vi "dat_muxed_thermistors.vi"() -> (20 "v_piston_0":fxp<+/-,24,5>, 21 "v_piston_1":fxp<+/-,24,5>, 22 "v_piston_2":fxp<+/-,24,5>, 23 "v_piston_3":fxp<+/-,24,5>, 24 "v_piston_4":fxp<+/-,24,5>, 25 "v_piston_5":fxp<+/-,24,5>, 26 "v_piston_6":fxp<+/-,24,5>, 27 "v_piston_7":fxp<+/-,24,5>)   [LabVIEW 2018]
uses:
  <vilib>/rvi/DataTransferAndStorage/Container/Common/niFpgaContainerExecOnDevCompGetState.vi
  <vilib>/rvi/Emulation/niFpgaEmulationIsFPGAContextNoSignature.vi
  <vilib>/rvi/Emulation/niFpgaSctlEmulationGetInTimedLoop.vi
  <vilib>/rvi/errors/niFpgaSetErrorForExecOnDevCompSimple.vi
  <vilib>/rvi/eio/common/nirviEmuReportErrorAndStop.vi
  <vilib>/rvi/DataTransferAndStorage/Container/Common/niFpgaContainerGetUniqueNameForEmu.vi
  <vilib>/rvi/FIFO/Fifo_Resource/nirvififoEmulationSetSize.vi
  <vilib>/rvi/FIFO/Fifo_Resource/nirviFifoEmulationQueueMgr.vi
  <instcachedir>/0/nirviFifoEmulationQueueMgr_E5CAEC123FF24DC58D834DCA3CDAA9B5.lvgen/nirviFifoEmulationQueueMgr_E5CAEC123FF24DC58D834DCA3CDAA9B5_003.vi
  <vilib>/rvi/FIFO/Fifo_Resource/nirvififoEmulationDetermineInputValidOut.vi
  <vilib>/rvi/FIFO/Fifo_Resource/nirvififoEmulationCreateLock.vi
  <vilib>/rvi/Emulation/niFpgaProcessEmulError.vi
  <vilib>/rvi/FIFO/Fifo_Resource/nirvififoEmulationObtainLock.vi
  <vilib>/rvi/FIFO/Fifo_Resource/nirvififoEmulationReleaseLock.vi
  <vilib>/rvi/occurrence/nirviWaitOnOccurrenceBase.vi
  <vilib>/rvi/errors/nirviReportUnexpectedCaseInternalError.vi
  <vilib>/rvi/errors/nirviReportUnexpectedCaseInternalError (U32).vi
  <vilib>/Utility/error.llb/Clear Errors.vi
  <vilib>/rvi/interface/RandomDataEmulation/niFpgaRandomDataHandleErrors.vi
  <vilib>/rvi/DataTransferAndStorage/Container/XNode/niFpgaContainer.xnode
  <vilib>/rvi/FIFO/Fifo_Resource/niFpgaFifoEmulationRefIn.vi
types:
  T1 = cluster{"Analog":fxp<+/-,24,5>, "Index":fxp<+,3,3>}
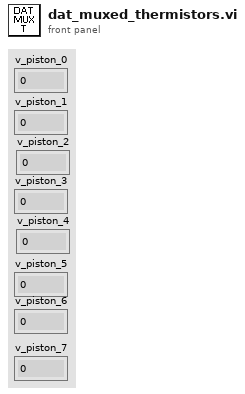
[diagram p1: front panel]
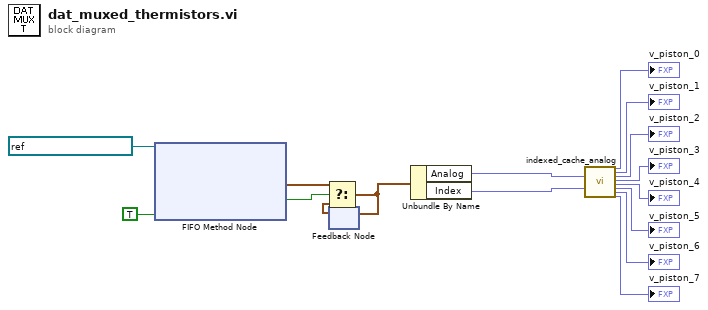
[diagram p0: block diagram]
diagram:
  n1 = xnode ("FIFO Method Node")("Ready for Output"=TRUE, "FIFO In"=refnum<k21> "T_pistons_indexed") -> ("Element"=w3:T1, "Output Valid"=w4:bool)  [unwired: 1 out]
  n2 = feedback #1() -> (w1:T1)  [unwired: 1 in]
  n3 = Select(t=w3, s=w4, f=w1) -> (s? t:f=w2:T1)
  n4 = feedback-in #1(w2) -> ()
  n5 = Unbundle By Name(w2) -> ("Analog"=w16:fxp<+/-,24,5>, "Index"=w15:fxp<+,3,3>)
  n6 = call "indexed_cache_analog.vi"("new_val"=w16, "index"=w15) -> ("$val_0"=→"v_piston_0":fxp<+/-,24,5>, "$val_1"=→"v_piston_1":fxp<+/-,24,5>, "$val_2"=→"v_piston_2":fxp<+/-,24,5>, "$val_3"=→"v_piston_3":fxp<+/-,24,5>, "$val_4"=→"v_piston_4":fxp<+/-,24,5>, "$val_5"=→"v_piston_5":fxp<+/-,24,5>, "$val_6"=→"v_piston_6":fxp<+/-,24,5>, "$val_7"=→"v_piston_7":fxp<+/-,24,5>)  [unwired: 18 in]
